vi "RINSE.vi"(11 "LWSR":refnum<class "Web Request.lvclass">) -> (0 "Temp (C) 2":dbl, 1 "Cond (mS) 2":dbl, 2 "Temp (C)":dbl, 3 "Cond (mS)":dbl, 4 "start_time":string, 6 "end_time":string, 8 "GUID":string)   [LabVIEW 2019]
uses:
  <vilib>/wsapi/Web Request.lvclass
  <vilib>/Utility/file.llb/Read Delimited Spreadsheet (string).vi
  <vilib>/Utility/file.llb/Write Delimited Spreadsheet (DBL).vi
panel:
  in  "Vacuum?":bool
  out "ViscoIteration":i32
  out "waste valve":string
  out "open valve":string
  out "Open-Air Valve#":i32
  out "Rinse Solvent Valve#":i32
  out "Chemical, volume (uL) ,valve position":string[][](array[string])=[["", "", "", "30"]]
  out "Splits":i32=4
  out "Constituents":i32=1
  out "run type":string
  out "run ID":string
  out "run order":string
  out "inventory":string
  out "postdata":string
  out "request method":string
  out "request URI":string
  out "content type":string
  out "remote address":string
  out "Hz":dbl
  out "Pump2_uL/stroke_":i32
  out "Pump1_uL/stroke_":i32
  in  "Pump2_uL/stroke":i32=6
  in  "Pump1_uL/stroke":i32=5
  out "Temp_Calib_Offset":dbl=4.8
  out "Cell_Constant":dbl=0.4
  out "RPM":i32
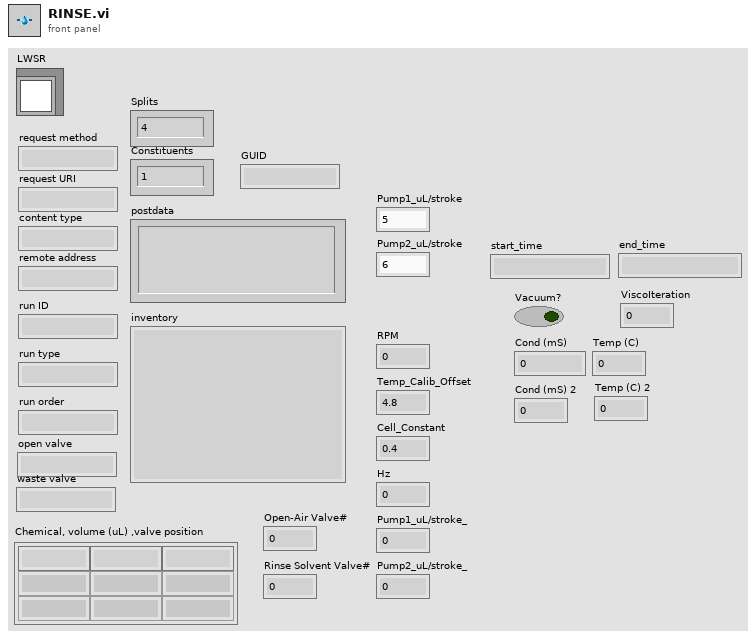
[diagram p1: front panel]
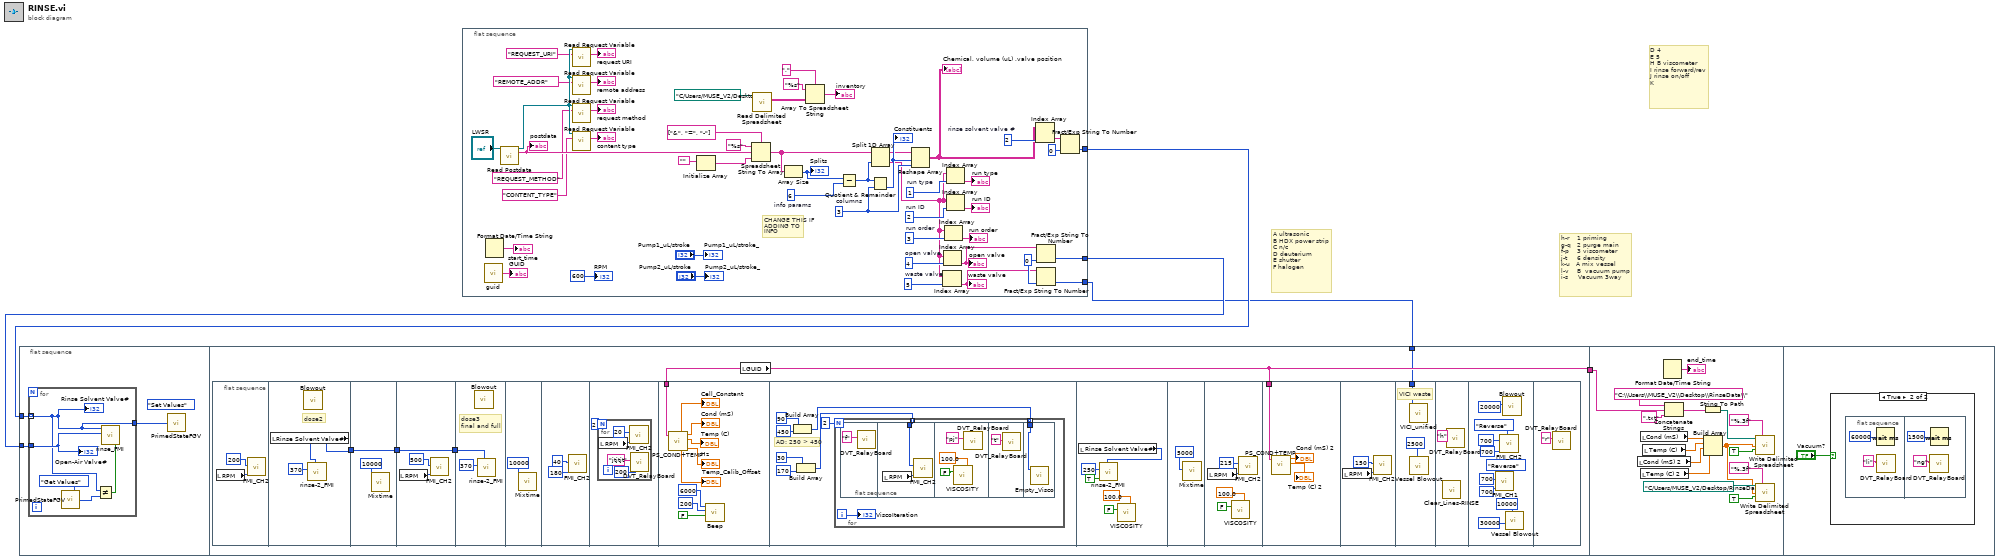
[diagram p0: block diagram]
diagram:
  # "h-r    1 priming\ng-q   2 purge main\nf-p    3 viscometer\nj-t     6 density\nk-u   A mix vessel\nl-v    B  vacuum pump\ni-s     Vacuum 3way"
  # "D 4 \nE 5 \nH B viscometer\nI rinse forward/rev\nJ rinse on/off\nK"
  # "A ultrasonic\nB HDX power strip\nC n/c\nD deuterium\nE shutter\nF halogen"
  n1 = flat-sequence {
    tunnel: w2 -> [w6]
    tunnel: w3 -> [w7]
    tunnel: [w16] -> w4
    tunnel: w1 -> [w13]
    tunnel: w4 -> [w102]
    frame #0 {
      (unwired) enum16{"Set Values", "Set Time", "Get Values"}."Set Values" ("Enum")
      n2 = for {
        tunnel: w6 -> [w8] mode=indexing
        tunnel: w7 -> [w12]
        tunnel: [w8] -> w5
        n3 = call "PrimedStateFGV.vi"("Enum"=enum16{"Set Values", "Set Time", "Get Values"}."Get Values") -> ("LastValve_read"=w11:i32)  [unwired: 13 in, 1 out]
        n4 = Not Equal?(x=w8, y=w11) -> (x != y?=w9:bool)
        n5 = call "rinse_FMI.vi"("Prime?"=w9, "OpenValve#"=w12, "RequestedValve#"=w8) -> ()  [unwired: 5 in]
        "Rinse Solvent Valve#" <- w8
        "Open-Air Valve#" <- w12
      }
      n6 = call "PrimedStateFGV.vi"("LastValve_write"=w5) -> ()  [unwired: 13 in, 2 out]
    }
    frame #1 {
      n7 = flat-sequence {
        tunnel: [w20] -> w15
        tunnel: w15 -> [w23]
        tunnel: [w23] -> w14
        tunnel: [w24] -> w17
        tunnel: w14 -> [w24]
        tunnel: w17 -> [w27]
        tunnel: w16 -> [w40]
        tunnel: w16 -> [w76]
        tunnel: w13 -> [w79]
        frame #0 {
          n8 = local read "RPM"() -> (w18:i32)
          n9 = call "FMI_CH2.vi"("RPM"=w18, "Strokes"=200) -> ()  [unwired: 5 in, 1 out]
        }
        frame #1 {
          # "dose2"
          n10 = local read "Rinse Solvent Valve#"() -> (w20:i32)
          n11 = call "Blowout.vi"() -> ()  [unwired: 12 in]
          n12 = call "rinse-2_FMI.vi"("RequestedValve#"=w20, "Strokes"=370) -> ()  [unwired: 10 in]
        }
        frame #2 {
          n13 = call "Mixtime.vi"("Mixtime(ms)"=u32 10000) -> ()  [unwired: 11 in]
        }
        frame #3 {
          n14 = local read "RPM"() -> (w26:i32)
          n15 = call "FMI_CH2.vi"("RPM"=w26, "Strokes"=500) -> ()  [unwired: 5 in, 1 out]
        }
        frame #4 {
          # "dose3\nfinal and full"
          n16 = call "Blowout.vi"() -> ()  [unwired: 12 in]
          n17 = call "rinse-2_FMI.vi"("RequestedValve#"=w27, "Strokes"=370) -> ()  [unwired: 10 in]
        }
        frame #5 {
          n18 = call "Mixtime.vi"("Mixtime(ms)"=u32 10000) -> ()  [unwired: 11 in]
        }
        frame #6 {
          n19 = call "FMI_CH2.vi"("RPM"=180, "Strokes"=40) -> ()  [unwired: 5 in, 1 out]
        }
        frame #7 {
          n20 = for {
            N: 2 -> [_]
            n21 = local read "RPM"() -> (w34:i32)
            n22 = call "FMI_CH2.vi"("RPM"=w34, "Strokes"=20) -> ()  [unwired: 5 in, 1 out]
            n23 = call "DVT_RelayBoard.vi"("ms"=u32 200, "write buffer"="jtjtjt") -> ()  [unwired: 2 in, 3 out]
          }
        }
        frame #8 {
          n24 = call "PS_COND+TEMP.vi"("GUID"=w40) -> ("Cell_Constant"=→"Cell_Constant":dbl, "Cond (mS)"=→"Cond (mS)":dbl, "Temp (C)"=→"Temp (C)":dbl, "Temp_Calib_Offset"=→"Temp_Calib_Offset":dbl, "Hz"=→"Hz":dbl)  [unwired: 1 in, 4 out]
          n25 = call <vilib>:"Beep.vi"("use system alert? (T)"=FALSE, "duration (msec)"=u32 200, "frequency (Hz)"=u32 6000) -> ()  [unwired: 9 in]
        }
        frame #9 {
          # "AD: 250 > 450"
          n26 = Build Array(90, 450) -> (w52:i32[])
          n27 = Build Array(30, 170) -> (w51:i32[])
          n28 = for {
            N: 2 -> [_]
            tunnel: w51 -> [w55] mode=indexing
            tunnel: w52 -> [w54] mode=indexing
            i -> [w53]
            n29 = flat-sequence {
              tunnel: w55 -> [w57]
              tunnel: w54 -> [w63]
              frame #0 {
                n30 = call "DVT_RelayBoard.vi"("write buffer"="f") -> ()  [unwired: 3 in, 3 out]
              }
              frame #1 {
                n31 = local read "RPM"() -> (w58:i32)
                n32 = call "FMI_CH2.vi"("RPM"=w58, "Strokes"=w57) -> ()  [unwired: 5 in, 1 out]
              }
              frame #2 {
                n33 = call "VISCOSITY.vi"("Startup RPM"=100.0, "LogData? (T)"=FALSE ("LogData?")) -> ()  [unwired: 7 in, 7 out]
                n34 = call "DVT_RelayBoard.vi"("write buffer"="pj") -> ()  [unwired: 3 in, 3 out]
              }
              frame #3 {
                n35 = call "DVT_RelayBoard.vi"("write buffer"="t") -> ()  [unwired: 3 in, 3 out]
              }
              frame #4 {
                n36 = call "Empty_Visco.vi"("Strokes"=w63) -> ()  [unwired: 11 in]
              }
            }
            "ViscoIteration" <- w53
          }
        }
        frame #10 {
          n37 = local read "Rinse Solvent Valve#"() -> (w66:i32)
          n38 = call "rinse-2_FMI.vi"("RequestedValve#"=w66, "Last?"=TRUE, "Strokes"=250) -> ()  [unwired: 9 in]
          n39 = call "VISCOSITY.vi"("Startup RPM"=100.0, "LogData? (T)"=FALSE ("LogData?")) -> ()  [unwired: 7 in, 7 out]
        }
        frame #11 {
          n40 = call "Mixtime.vi"("Mixtime(ms)"=u32 5000) -> ()  [unwired: 11 in]
        }
        frame #12 {
          n41 = local read "RPM"() -> (w73:i32)
          n42 = call "VISCOSITY.vi"("Startup RPM"=100.0, "LogData? (T)"=FALSE ("LogData?")) -> ()  [unwired: 7 in, 7 out]
          n43 = call "FMI_CH2.vi"("RPM"=w73, "Strokes"=215) -> ()  [unwired: 5 in, 1 out]
        }
        frame #13 {
          n44 = call "PS_COND+TEMP.vi"("GUID"=w76) -> ("Cond (mS)"=→"Cond (mS) 2":dbl, "Temp (C)"=→"Temp (C) 2":dbl)  [unwired: 1 in, 7 out]
        }
        frame #14 {
          n45 = local read "RPM"() -> (w77:i32)
          n46 = call "FMI_CH2.vi"("RPM"=w77, "Strokes"=150) -> ()  [unwired: 5 in, 1 out]
        }
        frame #15 {
          # "VICI waste"
          n47 = call "VICI_unified.vi"("RequestedValve#"=w79) -> ()  [unwired: 11 in]
          n48 = call "Vessel Blowout.vi"("Blowtime(ms)"=u32 2500 ("Mixtime(ms)")) -> ()  [unwired: 11 in]
        }
        frame #16 {
          n49 = call "Clear_Lines-RINSE.vi"() -> ()  [unwired: 12 in]
          n50 = call "DVT_RelayBoard.vi"("write buffer"="h") -> ()  [unwired: 3 in, 3 out]
        }
        frame #17 {
          n51 = call "FMI_CH1.vi"("Direction"=enum16{"Forward", "Reverse"}."Reverse", "RPM"=700, "Strokes"=700) -> ()  [unwired: 5 in]
          n52 = call "FMI_CH2.vi"("Direction"=enum16{"Forward", "Reverse"}."Reverse", "RPM"=700, "Strokes"=700) -> ()  [unwired: 4 in, 1 out]
          n53 = call "Blowout.vi"("Blowout (ms)"=u32 20000) -> ()  [unwired: 11 in]
          n54 = call "Vessel Blowout.vi"("Blowtime(ms)"=u32 10000 ("Mixtime(ms)"), "Delay(ms)"=u32 30000) -> ()  [unwired: 10 in]
        }
        frame #18 {
          n55 = call "DVT_RelayBoard.vi"("write buffer"="r") -> ()  [unwired: 3 in, 3 out]
        }
      }
      n56 = local read "GUID"() -> (w16:string)
    }
    frame #2 {
      n57 = local read "Cond (mS) 2"() -> (w93:dbl)
      n58 = local read "Cond (mS)"() -> (w99:dbl)
      n59 = local read "Temp (C) 2"() -> (w92:dbl)
      n60 = local read "Temp (C)"() -> (w100:dbl)
      n61 = Format Date/Time String() -> (date/time string=→"end_time":string)  [unwired: 3 in]
      n62 = Concatenate Strings("C:\\Users\\MUSE_V2\\Desktop\\RinseData\\", w102, ".txt" ("string")) -> (w104:string)
      n63 = String To Path(string=w104) -> (path=w101:path)
      n64 = Build Array(w99, w100, w93, w92) -> (w94:dbl[])
      n65 = call-poly <vilib>:"Write Delimited Spreadsheet.vi"("file path (dialog if empty)"=w101, "format (%.3f)"="%.3f", "1D data"=w94, "append to file? (new file:F)"=TRUE) -> ()  [unwired: 10 in, 2 out]
      n66 = call-poly <vilib>:"Write Delimited Spreadsheet.vi"("file path (dialog if empty)"=path "C:/Users/MUSE_V2/Desktop/RinseData/01_AppendedLog.txt" ("file path (use dialog)"), "format (%.3f)"="%.3f", "1D data"=w94, "append to file? (new file:F)"=TRUE) -> ()  [unwired: 10 in, 2 out]
    }
    frame #3 {
      n67 = case shown="True" "Vacuum?" {
        frame False {
        }
        frame True {
          n68 = flat-sequence {
            frame #0 {
              n69 = Wait (ms)(milliseconds to wait=u32 60000) -> ()  [unwired: 1 out]
              n70 = call "DVT_RelayBoard.vi"("write buffer"="li") -> ()  [unwired: 3 in, 3 out]
            }
            frame #1 {
              n71 = call "DVT_RelayBoard.vi"("write buffer"="ng") -> ()  [unwired: 3 in, 3 out]
              n72 = Wait (ms)(milliseconds to wait=u32 1500) -> ()  [unwired: 1 out]
            }
          }
        }
      }
    }
  }
  n73 = flat-sequence {
    tunnel: [w163] -> w3
    tunnel: [w159] -> w2
    tunnel: [w113] -> w1
    frame #0 {
      w117 = 5  # waste valve
      w115 = 0 ("default (0 DBL)")
      w124 = 4  # open valve
      w144 = 3  # run order
      w147 = 2  # run ID
      w148 = 1  # run type
      w150 = 6  # info params
      w154 = 3  # columns
      w162 = 2  # rinse solvent valve #
      # "CHANGE THIS IF\nADDING TO \nINFO"
      n74 = call "guid.vi"() -> ("GUID String"=→"GUID":string)  [unwired: 1 in]
      n75 = Format Date/Time String() -> (date/time string=→"start_time":string)  [unwired: 3 in]
      n76 = call <vilib>:"Read Postdata.vi"("LabVIEW Web Service Request"="LWSR") -> ("LabVIEW Web Service Request out"=w131:refnum<class "Web Request.lvclass">, "postdata"=w137:string)  [unwired: 12 in, 1 out]
      "postdata" <- w137
      n77 = call <vilib>:"Read Request Variable.vi"("LabVIEW Web Service Request"=w131, "variable name"="REQUEST_URI" ("request uri")) -> ("value"=→"request URI":string)  [unwired: 11 in, 2 out]
      n78 = call <vilib>:"Read Request Variable.vi"("LabVIEW Web Service Request"=w131, "variable name"="REMOTE_ADDR" ("remote address")) -> ("value"=→"remote address":string)  [unwired: 11 in, 2 out]
      n79 = call <vilib>:"Read Request Variable.vi"("LabVIEW Web Service Request"=w131, "variable name"="REQUEST_METHOD" ("request method")) -> ("value"=→"request method":string)  [unwired: 11 in, 2 out]
      n80 = call <vilib>:"Read Request Variable.vi"("LabVIEW Web Service Request"=w131, "variable name"="CONTENT_TYPE" ("content type")) -> ("value"=→"content type":string)  [unwired: 11 in, 2 out]
      n81 = Initialize Array("") -> (w156:string[])  [unwired: 1 in]
      n82 = Spreadsheet String To Array(delimiter (Tab)=string[] ["&", "=", "-"], format string="%s", spreadsheet string=w137, array type (2D Dbl)=w156) -> (array=w149:string[])
      n83 = call-poly <vilib>:"Read Delimited Spreadsheet.vi"("file path (dialog if empty)"=path "C:/Users/MUSE_V2/Desktop/CLIO/Public Content/inventory.csv") -> ("all rows"=w141:string[][])  [unwired: 9 in, 5 out]
      n84 = Array Size(array=w149) -> (size(s)=w151:i32)
      "Splits" <- w151
      n85 = Array To Spreadsheet String(delimiter (Tab)=",", array=w141, 3:"%s" ("format string")) -> (spreadsheet string=→"inventory":string)
      n86 = Subtract(x=w151, y=w150) -> (x-y=w136:i32)
      n87 = Split 1D Array(array=w149, index=w136) -> (first subarray=w142:string[], second subarray=w116:string[])
      n88 = Quotient & Remainder(x=w136, y=w154) -> (floor(x/y)=w153:i32)  [unwired: 1 out]
      "Constituents" <- w153
      n89 = Reshape Array(w142, w153, w154) -> (w161:string[][])
      "Chemical, volume (uL) ,valve position" <- w161
      n90 = Index Array(array=w116, index=w117) -> (element=w114:string)
      "waste valve" <- w114
      n91 = Index Array(array=w116, index=w124) -> (element=w123:string)
      "open valve" <- w123
      n92 = Index Array(array=w116, index=w144) -> (element=→"run order":string)
      n93 = Index Array(array=w116, index=w148) -> (element=→"run type":string)
      n94 = Index Array(array=w116, index=w147) -> (element=→"run ID":string)
      n95 = Index Array(array=w161, index (col)=w162) -> (element=w160:string[])  [unwired: 1 in]
      n96 = Fract/Exp String To Number(string=w123, default (0 dbl)=w115) -> (number=w163:i32)  [unwired: 2 in, 1 out]
      n97 = Fract/Exp String To Number(string=w114, default (0 dbl)=w115) -> (number=w113:i32)  [unwired: 2 in, 1 out]
      n98 = Fract/Exp String To Number(string=w160, default (0 dbl)=0 ("default (0 DBL)")) -> (number=w159:i32[])  [unwired: 2 in, 1 out]
      "RPM" <- 600
      "Pump1_uL/stroke_" <- "Pump1_uL/stroke"
      "Pump2_uL/stroke_" <- "Pump2_uL/stroke"
    }
  }
